vi "Configure.vi"(8 "error in (no error)":errorcluster caption="错误输入（无错误）", 10 "Function":T1, 11 "DP 输入":refnum<class "DP.lvclass">) -> (0 "error out":errorcluster caption="错误输出", 3 "DP 输出":refnum<class "DP.lvclass">)   [LabVIEW 2020, in "DP.lvlib" / "DP.lvclass"]
uses:
  DP.lvclass
  DP.lvclass/DP.ctl
  Function.ctl
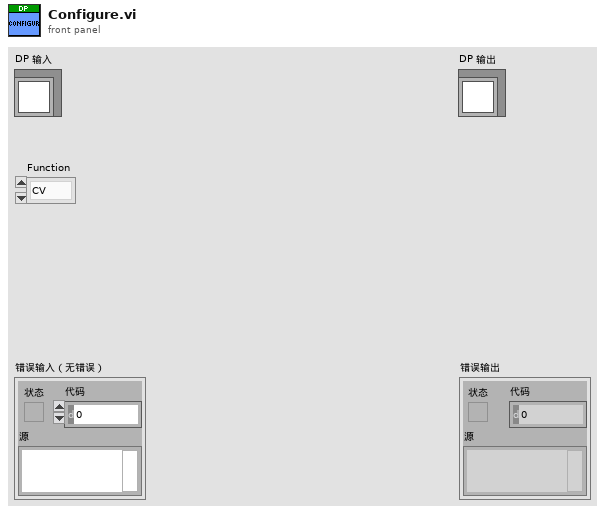
[diagram p1: front panel]
types:
  T1 = typedef "DP.lvlib/DP.lvclass/Function.ctl" = enum16{"CV", "CC"}
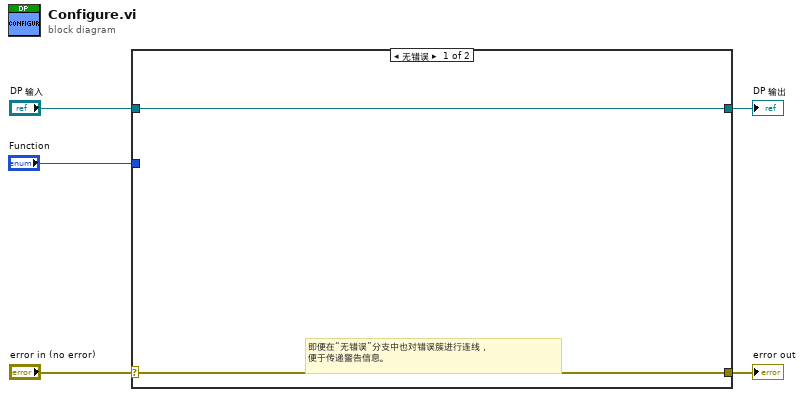
[diagram p0: block diagram]
diagram:
  n1 = case shown="无错误" "error in (no error)" {
    selector: "error in (no error)" -> [w6 w9]
    tunnel: [w6 w9] -> w4
    tunnel: [w7 w8] -> w2
    tunnel: "DP 输入" -> [w7 w8]
    tunnel: "Function" -> [_ _]
    frame No Error {
      # "即便在“无错误”分支中也对错误簇进行连线，\n便于传递警告信息。"
    }
    frame Error {
    }
  }
  "error out" <- w4
  "DP 输出" <- w2
